vi "Get HardDisk ID.vi"() -> ()   [LabVIEW 2013, in "ManagementClass.lvclass"]
uses:
  ManagementClass.lvclass
panel:
  out "Parameters":string[](array[string])
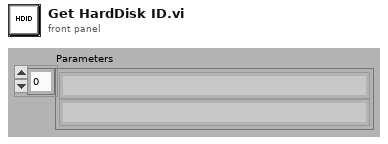
[diagram p1: front panel]
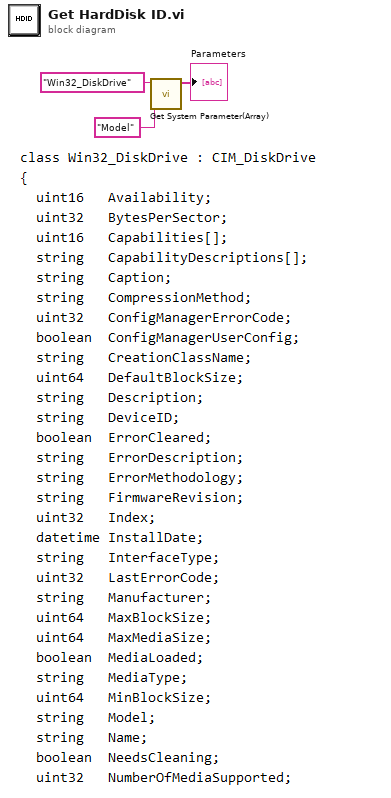
[diagram p0: block diagram]
diagram:
  n1 = call "Get System Parameter(Array).vi"("propertyName"="Model", "path"="Win32_DiskDrive") -> ("Parameters"=→"Parameters":string[])  [unwired: 8 in, 1 out]
